vi "Process Data2D.vi"(8 "error in (no error)":errorcluster, 10 "Data2D in":refnum<class "Data2D.lvclass">, 11 "AbstractProcessor2D in":refnum<class "AbstractProcessor2D.lvclass">) -> (0 "error out":errorcluster, 2 "Data2D out":refnum<class "Data2D.lvclass">, 3 "AbstractProcessor2D out":refnum<class "AbstractProcessor2D.lvclass">)   [LabVIEW 2014, in "AbstractProcessor2D.lvclass"]
uses:
  AbstractProcessor2D.lvclass
  Model/Data/Data2D/Data2D.lvclass
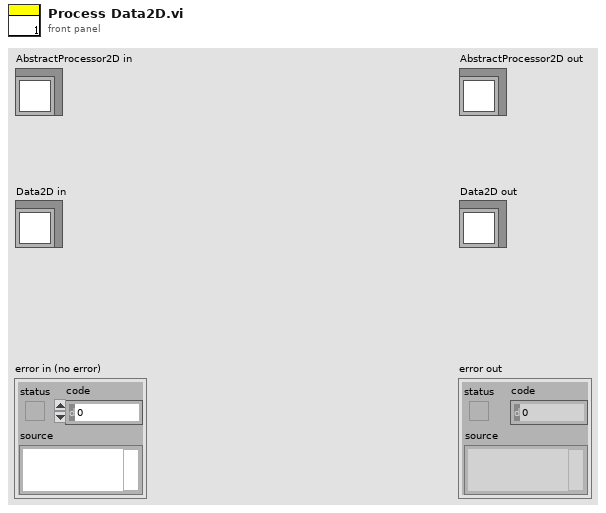
[diagram p1: front panel]
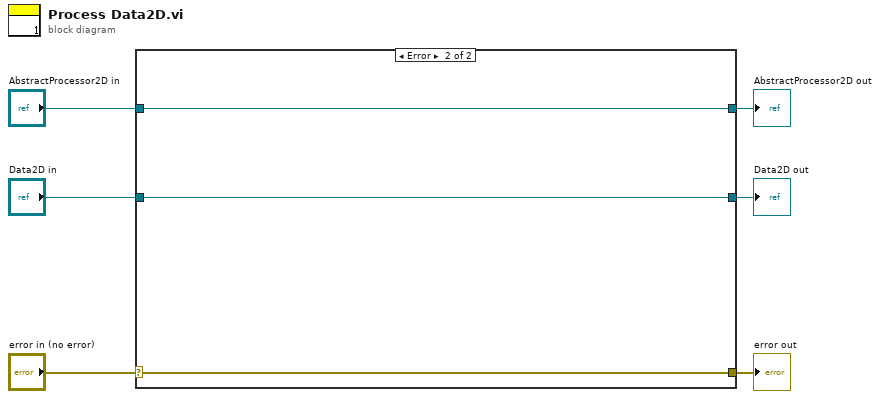
[diagram p0: block diagram]
diagram:
  n1 = case shown="Error" "error in (no error)" {
    selector: "error in (no error)" -> [w8 w12]
    tunnel: [w8 w12] -> w5
    tunnel: [w9 w11] -> w3
    tunnel: "AbstractProcessor2D in" -> [w9 w11]
    tunnel: [w7 w10] -> w2
    tunnel: "Data2D in" -> [w7 w10]
    frame No Error {
      # "Wire the error cluster across even in the \"No Error\"\ncase so that warnings get propagated."
    }
    frame Error {
    }
  }
  "error out" <- w5
  "AbstractProcessor2D out" <- w3
  "Data2D out" <- w2
